vi "SOURCE_CONFIG.vi"() -> ()   [LabVIEW 2020]
uses:
  <instrlib>/Agilent B2900 Series/Agilent B2900 Series.lvlib
panel:
  in  "VISA resource name":refnum<visa-resource-name>
  in  "error in (no error)":errorcluster
  out "VISA resource name out":refnum<visa-resource-name>
  out "error out":errorcluster
  in  "file path (use dialog)":path
  out "output string":string
  in  "Source Range Lower Limit (2 V)":dbl=2.0
  in  "Source Auto Range (T: Enable)":bool=TRUE
  in  "Channel (0: Channel 1)":i32(ring) items=["Channel 1", "Channel 2"]
  in  "Enable Continuous Output (T: Enable)":bool=TRUE
  in  "Source Range (2)":dbl=2.0
  in  "Source Shape (1: DC)":i32(ring)=1 items=["Pulse", "DC"]
  in  "Source Mode (1: Voltage)":i32(ring)=1 items=["Current", "Voltage"]
  in  "Triggered Output Level (0)":dbl
  in  "Output Level (0)":dbl
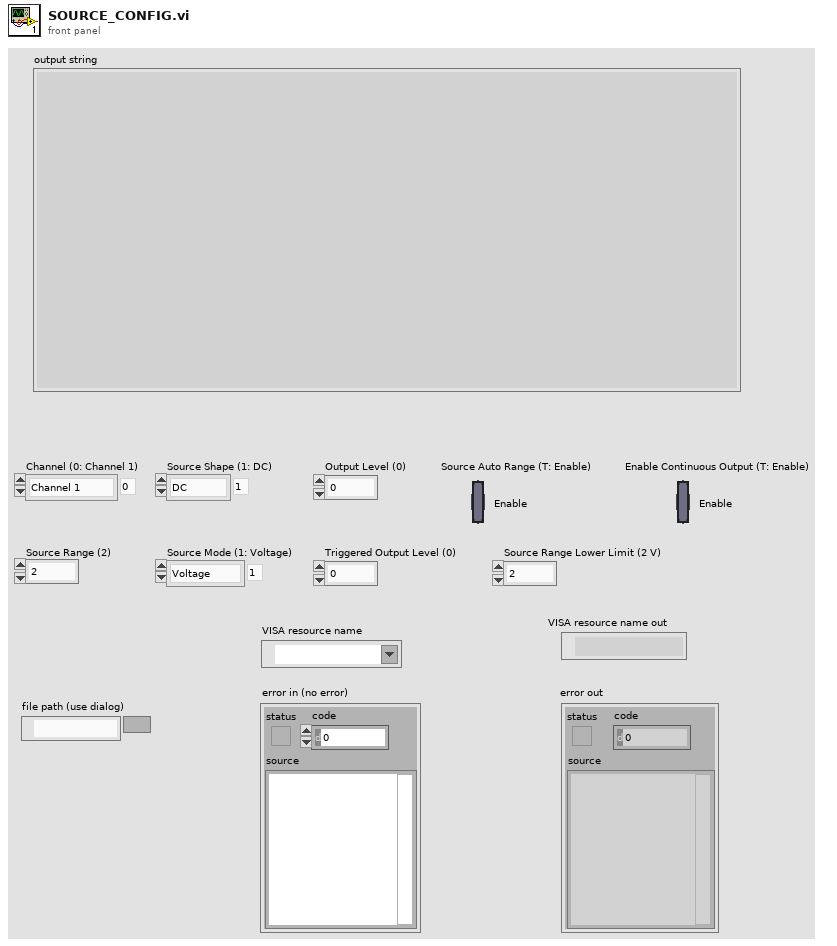
[diagram p1: front panel]
types:
  T1 = enum16{"open", "replace", "create", "open or create", "replace or create", "replace or create with confirmation"}
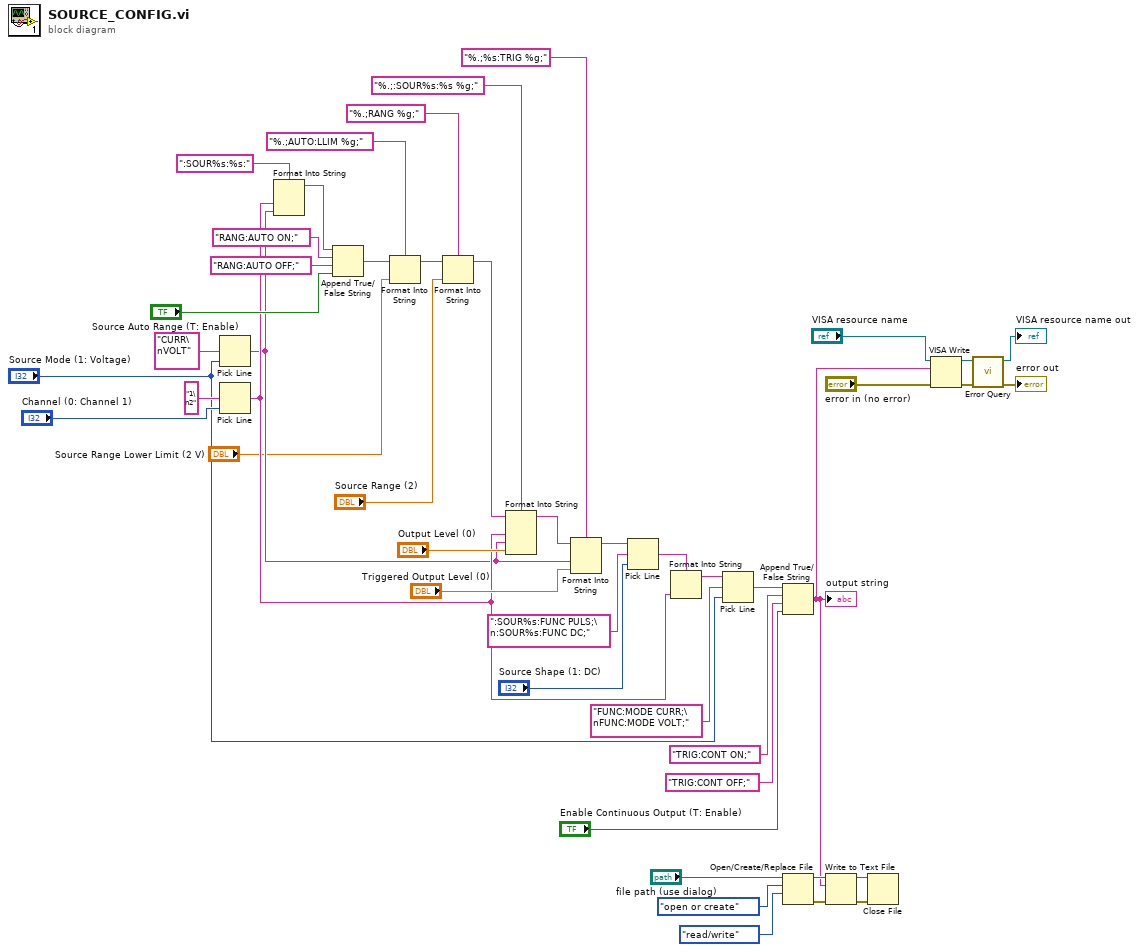
[diagram p0: block diagram]
diagram:
  n1 = Pick Line(multi-line string="CURR\nVOLT" ("string (\"\")"), line index="Source Mode (1: Voltage)") -> (output string=w21:string)  [unwired: 1 in]
  n2 = Pick Line(multi-line string="1\n2" ("string (\"\")"), line index="Channel (0: Channel 1)") -> (output string=w22:string)  [unwired: 1 in]
  n3 = Format Into String(format string=":SOUR%s:%s:", w22, w21) -> (resulting string=w19:string)  [unwired: 2 in, 1 out]
  n4 = Append True/False String(1:"Source Auto Range (T: Enable)", 2:"RANG:AUTO OFF;", 3:"RANG:AUTO ON;", 4:w19) -> (0:w16:string)
  n5 = Format Into String(format string="%.;AUTO:LLIM %g;", initial string=w16, "Source Range Lower Limit (2 V)") -> (resulting string=w18:string)  [unwired: 1 in, 1 out]
  n6 = Format Into String(format string="%.;RANG %g;", initial string=w18, "Source Range (2)") -> (resulting string=w28:string)  [unwired: 1 in, 1 out]
  n7 = Format Into String(format string="%.;:SOUR%s:%s %g;", initial string=w28, w22, w21, "Output Level (0)") -> (resulting string=w45:string)  [unwired: 1 in, 1 out]
  n8 = Format Into String(format string="%.;%s:TRIG %g;", initial string=w45, w21, "Triggered Output Level (0)") -> (resulting string=w27:string)  [unwired: 1 in, 1 out]
  n9 = Pick Line(string ("")=w27, multi-line string=":SOUR%s:FUNC PULS;\n:SOUR%s:FUNC DC;", line index="Source Shape (1: DC)") -> (output string=w35:string)
  n10 = Format Into String(format string=w35, w22) -> (resulting string=w34:string)  [unwired: 2 in, 1 out]
  n11 = Pick Line(string ("")=w34, multi-line string="FUNC:MODE CURR;\nFUNC:MODE VOLT;", line index="Source Mode (1: Voltage)") -> (output string=w33:string)
  n12 = Append True/False String(1:"Enable Continuous Output (T: Enable)", 2:"TRIG:CONT OFF;", 3:"TRIG:CONT ON;", 4:w33) -> (0:w1:string)
  "output string" <- w1
  n13 = Open/Create/Replace File(file path (use dialog)="file path (use dialog)", operation (0:open)=T1."open or create", access (0:read/write)=enum16{"read/write", "read-only", "write-only"}."read/write") -> (refnum out=w11:refnum<file>, error out=w9:errorcluster)  [unwired: 3 in, 1 out]
  n14 = Write to Text File(file (use dialog)=w11, text=w1, error in=w9) -> (refnum out=w10:refnum<file>, error out=w8:errorcluster)  [unwired: 1 in, 1 out]
  n15 = Close File(refnum=w10, error in=w8) -> ()  [unwired: 2 out]
  n16 = VISA Write(VISA resource name="VISA resource name", write buffer=w1, error in (no error)="error in (no error)") -> (VISA resource name out=w4:refnum<visa-resource-name>, error out=w5:errorcluster)  [unwired: 1 out]
  n17 = call <instrlib>:"Error Query.vi"("error in (no error)"=w5, "VISA resource name"=w4) -> ("error out"=→"error out":errorcluster, "VISA resource name out"=→"VISA resource name out":refnum<visa-resource-name>)  [unwired: 6 in, 2 out]
